vi "Build Order.vi"(8 "error in (no error)":errorcluster, 10 "Order Content":cluster{"Drink type":T1, "Options":T2[]}[](array[cluster]), 11 "Customer In":refnum<class "Customer.lvclass">) -> (0 "error out":errorcluster, 2 "Order Out":refnum<class "Order.lvclass">, 3 "Customer Out":refnum<class "Customer.lvclass">)   [LabVIEW 2020, in "Customer.lvclass"]
uses:
  Customer.lvclass
  C:/Program Files (x86)/National Instruments/LabVIEW 2020/vi.lib/Astemes/Triarc Framework/Process/Process.lvclass
  Support/Beverages/TypeDefs/Drink Type.ctl
  Support/Beverages/TypeDefs/Options.ctl
  Support/Order/Order.lvclass
  <vilib>/Astemes/Triarc Framework/Process/Process.lvclass
  Support/Beverages/Beverage/Beverage.lvclass
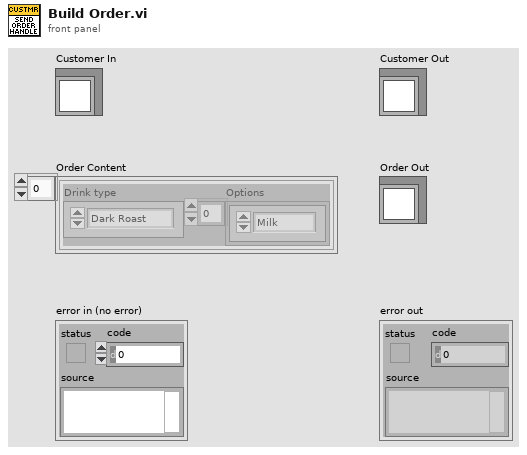
[diagram p1: front panel]
types:
  T1 = typedef "Beverage.lvclass/Drink Type.ctl" = enum16{"Dark Roast", "Decaf", "Espresso", "House Blend"}
  T2 = typedef "Beverage.lvclass/Options.ctl" = enum16{"<None>", "Milk", "Mocha", "Soy", "Whip"}
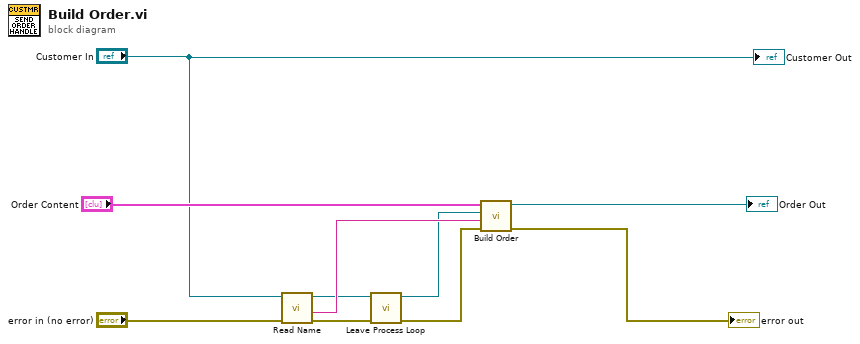
[diagram p0: block diagram]
diagram:
  n1 = call <vilib>:"Read Name.vi"("error in (no error)"="error in (no error)", "Process In"="Customer In") -> ("error out"=w2:errorcluster, "Name"=w8:string, "Process Out"=w4:refnum<class "Customer.lvclass">)  [unwired: 6 in, 1 out]
  n2 = call <vilib>:"Leave Process Loop.vi"("error in (no error)"=w2, "Process In"=w4) -> ("error out"=w1:errorcluster, "Process Out"=w3:refnum<class "Customer.lvclass">)  [unwired: 8 in]
  n3 = call "Build Order.vi"("error in (no error)"=w1, "Customer Name"=w8, "Customer"=w3, "Order"="Order Content") -> ("error out"=→"error out":errorcluster, "Order Out"=→"Order Out":refnum<class "Order.lvclass">)  [unwired: 6 in]
  "Customer Out" <- "Customer In"
